vi "VibratomeGUI.vi"(8 "Error Out":errorcluster, 11 "Remote?":bool) -> ()   [LabVIEW 2014]
uses:
  Hardware/Table Stage/Controls/Translation Stage Cluster.ctl
  Controls/Translation Stage Types.ctl
  Controls/Translation Stage Quick Status.ctl
  Controls/Translation Stage Quick Controls.ctl
  Controls/QueueNames.ctl
  Controls/Queue Manager Actions.ctl
  Controls/MessagePacket.ctl
  <vilib>/Utility/miscctls.llb/LVPointTypeDef.ctl
  Hardware/Table Stage/Controls/Motion Translation Module Control.ctl
  Controls/Set Get Controls.ctl
  Controls/FGV Actions.ctl
panel:
  in  "Z STEP MOTION":enum16{"Fine", "Course", "Extra Course"}(ring)
  in  "Stop Button":bool
  in  "Slice":bool
  in  "Vibratome Controls":T1
  out "Message":string
  in  "Z Ctrl":T2
  out "Z Status":T3
  in  "Y Ctrl":T2
  out "Y Status":T3
  in  "X Ctrl":T2
  out "X Status":T3
  in  "XY STEP MOTION":enum16{"Fine", "Course", "Extra Course"}(ring)
  out "Cluster":cluster{"X":T4, "Y":T4, "Z":T4}
  in  "Exit":bool
  out "Processor Error Out":errorcluster
  out "GUI Error Out":errorcluster
  # "Vibratome Controls"
  # "Z Axis"
  # "Y Axis"
  # "X Axis"
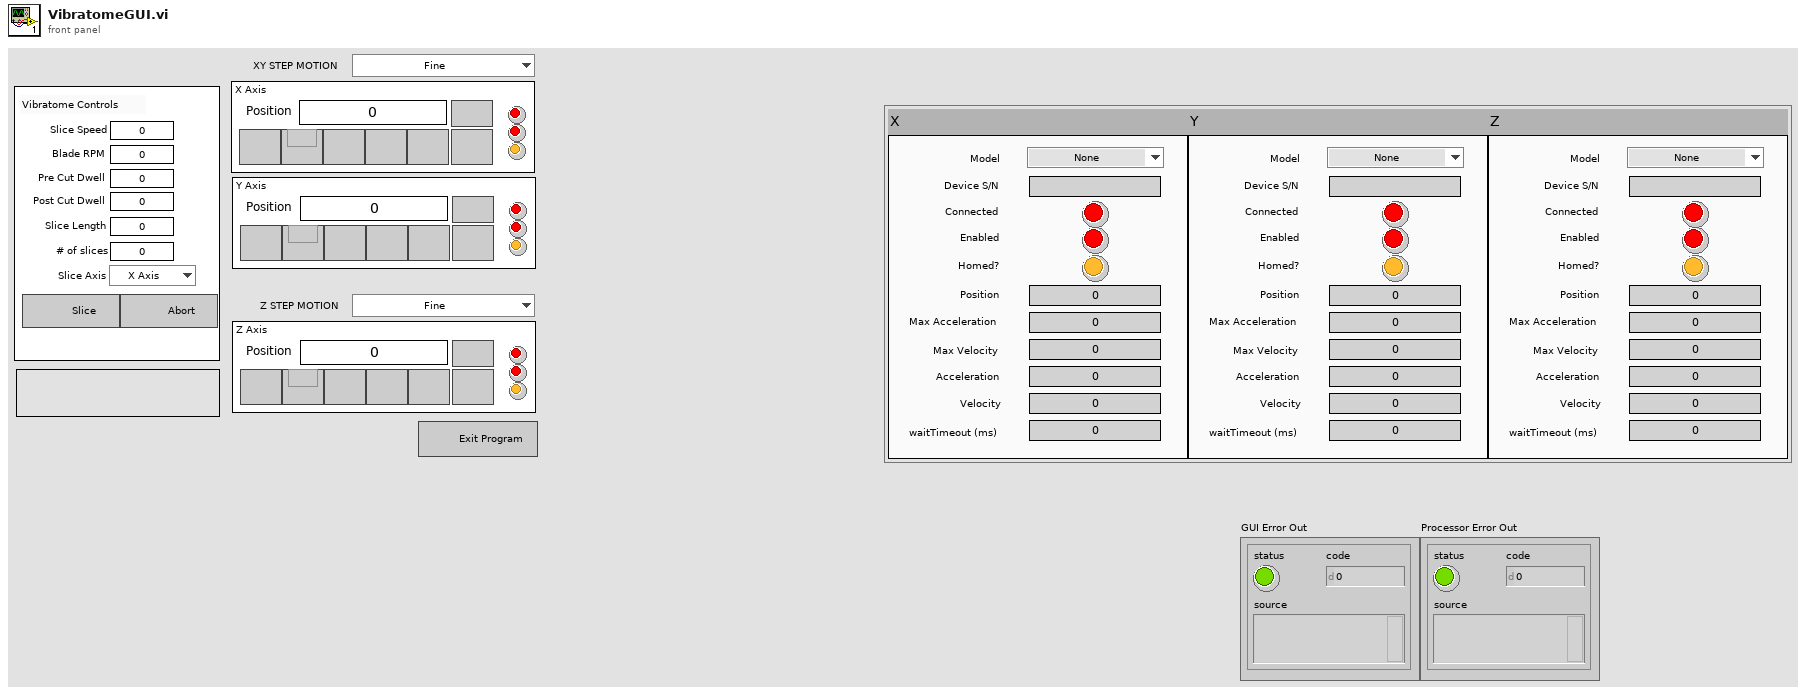
[diagram p1: front panel]
types:
  T1 = cluster{"Pre Cut Dwell":dbl, "Blade RPM":u16, "Slice Speed":dbl, "Post Cut Dwell":dbl, "Slice Length":dbl, "# of slices":dbl, "Slice Axis":enum16{"X Axis", "Y Axis", "Z Axis"}}
  T2 = typedef "Translation Stage Quick Controls.ctl" = cluster{"Position":dbl, "Next Button":bool, "Last Button":bool, "Previous Button":bool, "First Button":bool, "Home Button":bool, "Go":bool, "Settings Button":bool}
  T3 = typedef "Translation Stage Quick Status.ctl" = cluster{"Is.Enabled?":bool, "Is.Connected?":bool, "Is.Homed?":bool}
  T4 = typedef "Translation Stage Cluster.ctl" = cluster{"Position":dbl, "Is.Enabled?":bool, "Is.Connected?":bool, "Device SN":string, "AccelerationMaximum":dbl, "VelocityMaximum":dbl, "Acceleration":dbl, "Velocity":dbl, "waitTimeout (ms)":i32, "Model":T5, "Is.Homed?":bool}
  T5 = typedef "Translation Stage Types.ctl" = enum16{"None", "Thorlabs LTS", "Thorlabs MLJ"}
  T6 = typedef "MessagePacket.ctl" = cluster{"Message":string, "Parameter":variant}
  T7 = typedef "Queue Manager Actions.ctl" = enum16{"Init", "Enqueue", "Enqueue All", "Preview Queue", "Dequeue", "Get Status", "Flush Queue", "Flush All Queues", "Release All Queues", "Release Queue", "Enqueue at Opposite End"}
  T8 = typedef "QueueNames.ctl" = enum16{"Main GUI", "Main Scan Processor", "Main Display", "Main Table Stage GUI", "Main Table Stage Proc.", "Scan Engine", "Vibratome GUI", "Vibratome Processor", "Slice Engine"}
  T9 = enum16{"Set Configuration", "Get Configuration", "Enable Motor", "Disable Motor", "Get Status", "Open Session", "Close Session", "Set Limits", "Get Limits"}
  T10 = typedef "FGV Actions.ctl" = enum16{"Init", "Set", "Get", "Clear"}
  T11 = typedef "Set Get Controls.ctl" = enum16{"Set", "Get"}
  T12 = typedef "Motion Translation Module Control.ctl" = enum16{"Init", "Home", "Status", "Velocity/Accel", "Position", "Jog", "Stop", "Uninit", "Enable", "Disable"}
  T13 = cluster{"X Stage":T4, "Y Stage":T4, "Z Stage":T4}
  T14 = typedef "System Parameters.ctl" = cluster{"OCT":cluster{"Focal Length":dbl[unit]}, "Vibratome":cluster{"Z Bottom [mm]":dbl, "Pre Cut Dwell [s]":dbl, "Blade Frequency [RPM]":u16, "Slice Speed [mm/s]":dbl, "Post Cut Dwell [s]":dbl, "Ramp Time [s]":dbl, "Start X [mm]":dbl, "Start Y [mm]":dbl, "Slice Length [mm]":dbl, "Slice Axis":enum16{"X Axis", "Y Axis", "Z Axis"}, "Controller VISA Ref":refnum<visa-resource-name>}, "Table Stages":cluster{"X Stage":T4, "Y Stage":T4, "Z Stage":T4}}
  T15 = cluster{"Z Bottom [mm]":dbl, "Pre Cut Dwell [s]":dbl, "Blade Frequency [RPM]":u16, "Slice Speed [mm/s]":dbl, "Post Cut Dwell [s]":dbl, "Ramp Time [s]":dbl, "Start X [mm]":dbl, "Start Y [mm]":dbl, "Slice Length [mm]":dbl, "Slice Axis":enum16{"X Axis", "Y Axis", "Z Axis"}, "Controller VISA Ref":refnum<visa-resource-name>}
  T16 = enum32{"Invalid", "Default", "Floating", "Floating/Auto-Hide", "Modal"}
  T17 = enum32{"Invalid", "Standard", "Closed", "Hidden", "Minimized", "Maximized"}
  T18 = typedef "LVPointTypeDef.ctl" = cluster{"Horizontal":i16, "Vertical":i16}
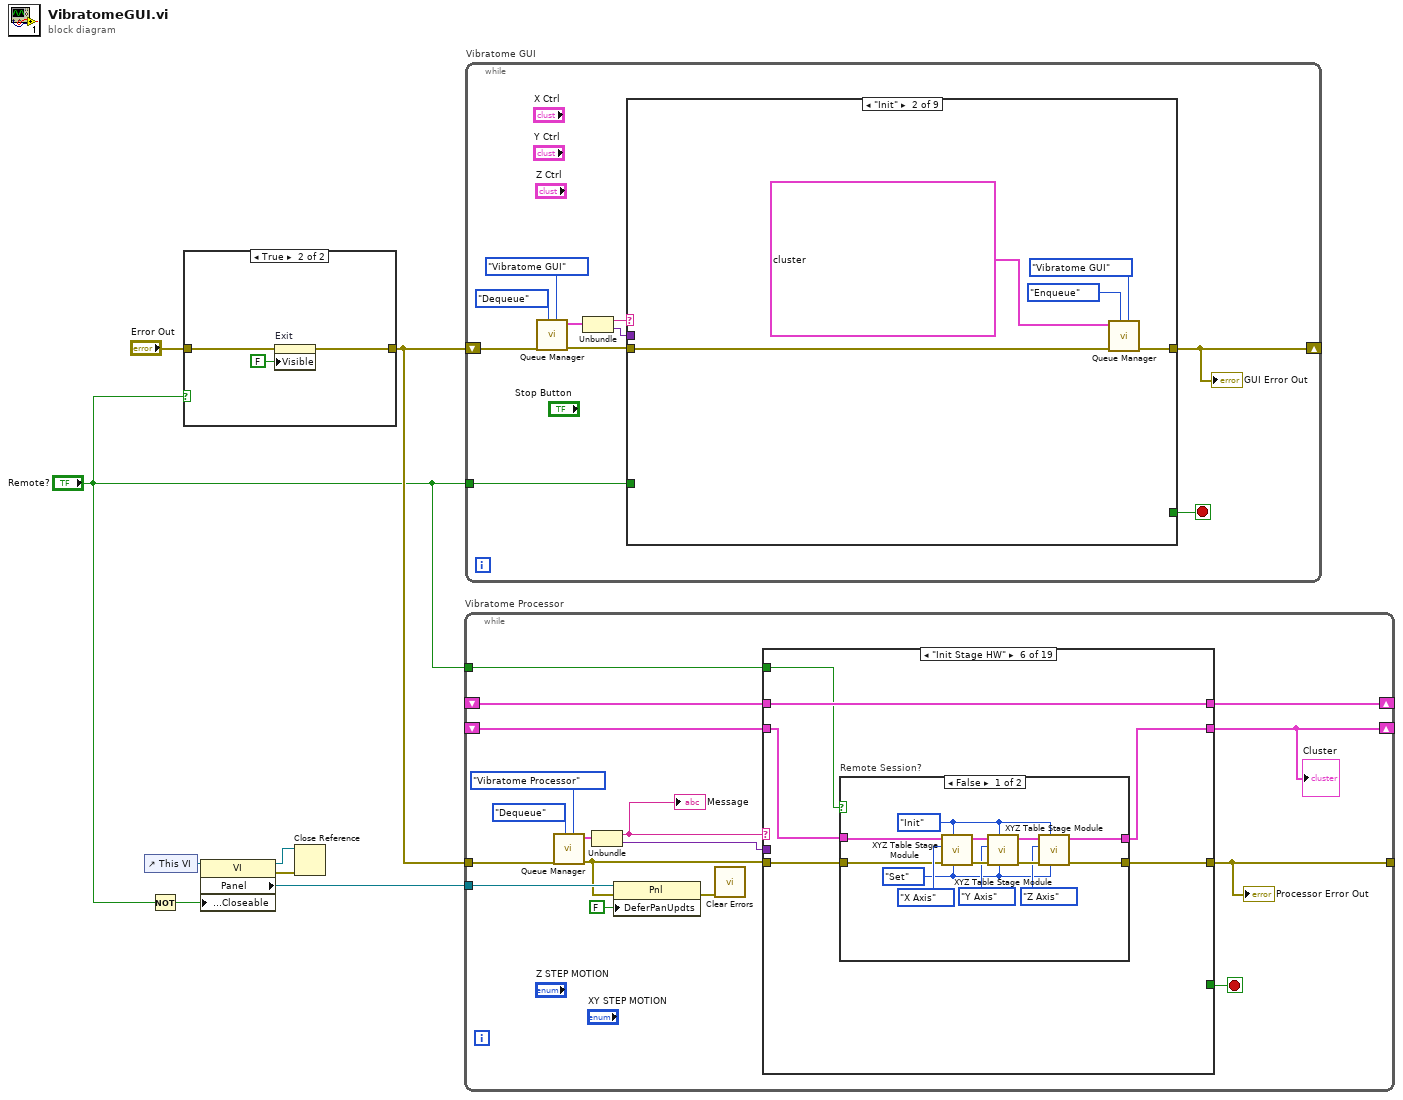
[diagram p0: block diagram]
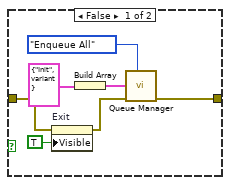
[diagram p2: hidden frame]
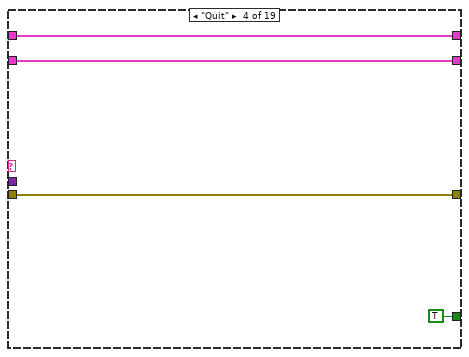
[diagram p6: hidden frame]
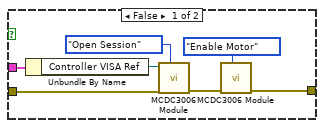
[diagram p10: hidden frame]
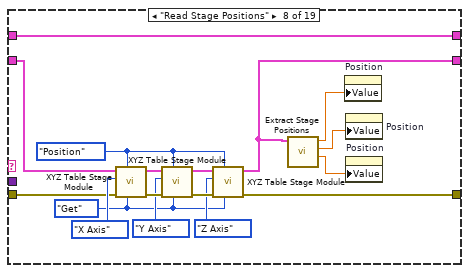
[diagram p11: hidden frame]
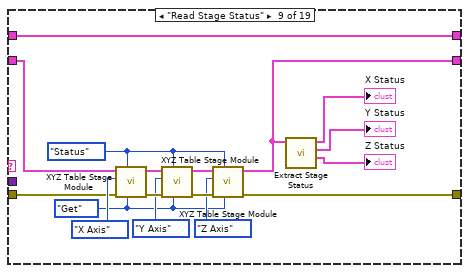
[diagram p12: hidden frame]
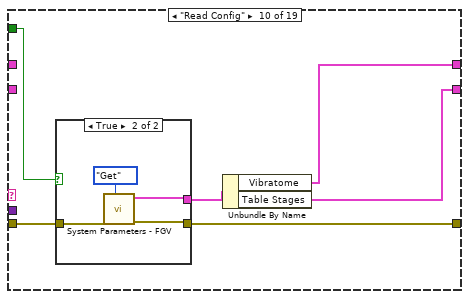
[diagram p13: hidden frame]
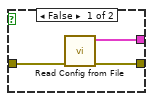
[diagram p14: hidden frame]
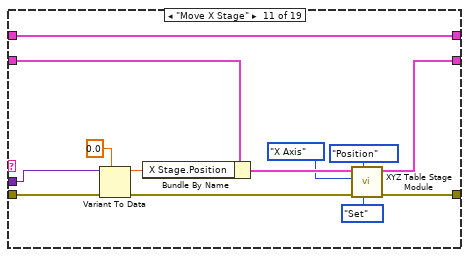
[diagram p15: hidden frame]
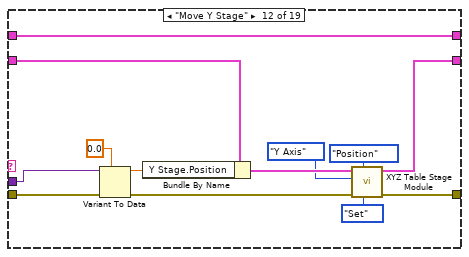
[diagram p16: hidden frame]
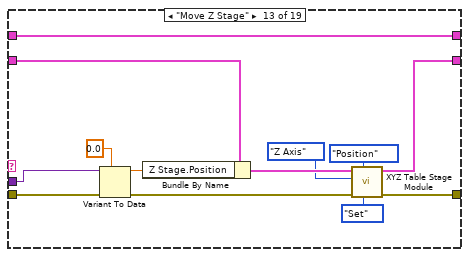
[diagram p17: hidden frame]
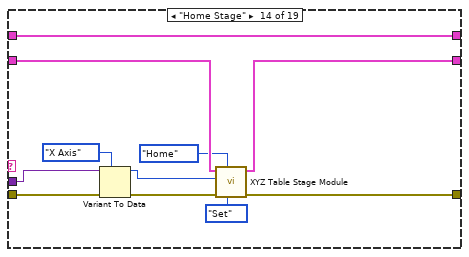
[diagram p18: hidden frame]
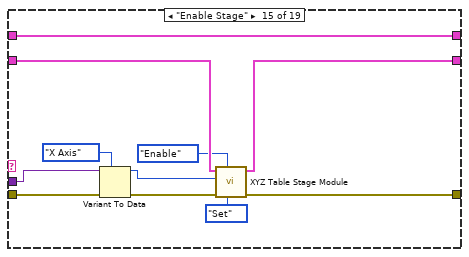
[diagram p19: hidden frame]
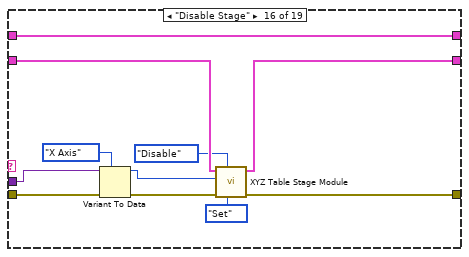
[diagram p20: hidden frame]
diagram:
  n1 = control-ref of="This VI"() -> (w7:refnum<vi>)
  n2 = Not(x="Remote?") -> (.not. x?=w1:bool)
  n3 = case shown="True" "Remote?" {
    tunnel: [w12 w17] -> w8
    tunnel: "Error Out" -> [w10 w18]
    frame False {
      n4 = property on="Exit" class="Bool"(error in=w10, "Visible"=TRUE) -> (error out=w9:errorcluster)  [unwired: 1 in, 1 out]
      n5 = Build Array(T6 {"Message"="Init", "Parameter"=variant} ("Message Packet [In]")) -> (w13:T6[])
      n6 = call "Queue Manager.vi"("Action"=Queue_Manager_Actions."Enqueue All", "Error In"=w9, "Message Packet Array"=w13) -> ("Error Out"=w12:errorcluster)  [unwired: 4 in, 4 out]
    }
    frame True {
      n7 = property on="Exit" class="Bool"(error in=w18, "Visible"=FALSE) -> (error out=w17:errorcluster)  [unwired: 1 in, 1 out]
    }
  }
  n8 = property class="VI"(reference=w7, "Front Panel.Closeable"=w1) -> (reference out=w5:refnum<vi>, error out=w6:errorcluster, "Panel"=w4:refnum<vi>)  [unwired: 1 in]
  n9 = Close Reference(reference=w5, error in (no error)=w6) -> ()  [unwired: 1 out]
  n10 = while "Vibratome Processor" {
    tunnel: w8 -> [w33]
    tunnel: [w35] -> _
    shift-right: [w24] -> _
    shift-left: _ -> [w27]
    shift-right: [w26] -> _
    shift-left: _ -> [w25]
    tunnel: w4 -> [w23]
    tunnel: "Remote?" -> [w19]
    stop <- w29 stop-if-true
    n11 = call "Queue Manager.vi"("Queue Name"=QueueNames."Vibratome Processor", "Action"=Queue_Manager_Actions."Dequeue", "Error In"=w33) -> ("Error Out"=w21:errorcluster, "Message Packet [Out]"=w32:T6)  [unwired: 4 in, 3 out]
    n12 = Unbundle(w32) -> ("Message"=w31:string, "Parameter"=w30:variant)
    "Message" <- w31
    n13 = property class="Pnl"(reference=w23, error in=w21, "DeferPanUpdts"=FALSE ("Defer Panel Updates")) -> (error out=w20:errorcluster)  [unwired: 1 out]
    n14 = call <vilib>:"Clear Errors.vi"("error in (no error)"=w20) -> ()  [unwired: 5 in, 2 out]
    n15 = case shown="\"Init Stage HW\"" w31 {
      tunnel: w21 -> [w38 w41 w42 w46 w49 w54 w74 w90 w107 w123 w143 w156 w169 w180 w191 w202 w207 w213 w233]
      tunnel: [w38 w41 w42 w46 w49 w55 w72 w98 w115 w121 w142 w155 w168 w179 w190 w201 w206 w212 w217] -> w35
      tunnel: w30 -> [_ _ _ _ _ _ _ _ _ _ w140 w153 w166 w177 w188 w199 _ _ _]
      tunnel: [_ _ _ TRUE _ _ _ _ _ _ _ _ _ _ _ _ _ _ _] -> w29
      tunnel: [w37 w40 w44 w48 _ w51 w75 w84 w105 w122 w139 w152 w165 w173 w184 w195 w204 w214 w226] -> w24
      tunnel: w27 -> [w37 w40 w44 w48 _ w53 w75 w89 w106 _ w135 w148 w161 w174 w185 w196 w204 w214 w229]
      tunnel: [w36 w39 w43 w47 _ w52 w73 w88 w101 w120 w131 w144 w157 w170 w181 w192 w208 w215 w220] -> w26
      tunnel: w25 -> [w36 w39 w43 w47 _ w52 w73 w88 w101 _ w131 w144 w157 w170 w181 w192 w208 w215 w220]
      tunnel: w19 -> [_ _ _ _ _ w50 w71 _ _ w118 _ _ _ _ _ _ _ _ _]
      frame "Unknown", Default {
      }
      frame "Finished Init" {
      }
      frame "Finished" {
      }
      frame "Quit" {
      }
      frame "Init" {
      }
      frame "Init Stage HW" {
        n16 = case "Remote Session?" shown="False" w50 {
          tunnel: [w66 w69] -> w55
          tunnel: w54 -> [w58 w69]
          tunnel: w53 -> [w57 w70]
          tunnel: [w56 w70] -> w51
          frame False {
            w59 = Set_Get_Controls."Set" ("Set/Get")
            w65 = Motion_Translation_Module_Control."Init" ("Action")
            n17 = call "XYZ Table Stage Module.vi"("Set/Get"=w59, "Action"=w65, "Error In"=w58, "Axis"=enum16{"X Axis", "Y Axis", "Z Axis"}."X Axis", "Table Stages"=w57) -> ("Error Out"=w68:errorcluster, "Table Stages Out"=w64:T13)  [unwired: 5 in]
            n18 = call "XYZ Table Stage Module.vi"("Set/Get"=w59, "Action"=w65, "Error In"=w68, "Axis"=enum16{"X Axis", "Y Axis", "Z Axis"}."Y Axis", "Table Stages"=w64) -> ("Error Out"=w67:errorcluster, "Table Stages Out"=w63:T13)  [unwired: 5 in]
            n19 = call "XYZ Table Stage Module.vi"("Set/Get"=w59, "Action"=w65, "Error In"=w67, "Axis"=enum16{"X Axis", "Y Axis", "Z Axis"}."Z Axis", "Table Stages"=w63) -> ("Error Out"=w66:errorcluster, "Table Stages Out"=w56:T13)  [unwired: 5 in]
          }
          frame True {
          }
        }
      }
      frame "Init Vibratome HW" {
        n20 = case "Remote Session?" shown="True" w71 {
          tunnel: w74 -> [w81 w83]
          tunnel: w73 -> [w79 _]
          tunnel: [w77 w83] -> w72
          frame False {
            n21 = Unbundle By Name(w79) -> ("Controller VISA Ref"=w78:refnum<visa-resource-name>)
            n22 = call "MCDC3006 Module.vi"("Actions"=T9."Open Session", "Error In"=w81, "VISA resource name"=w78) -> ("Error Out"=w80:errorcluster)  [unwired: 4 in, 4 out]
            n23 = call "MCDC3006 Module.vi"("Actions"=T9."Enable Motor", "Error In"=w80) -> ("Error Out"=w77:errorcluster)  [unwired: 5 in, 4 out]
          }
          frame True {
          }
        }
      }
      frame "Read Stage Positions" {
        w91 = Set_Get_Controls."Get" ("Set/Get")
        w97 = Motion_Translation_Module_Control."Position" ("Action")
        n24 = call "XYZ Table Stage Module.vi"("Set/Get"=w91, "Action"=w97, "Error In"=w90, "Axis"=enum16{"X Axis", "Y Axis", "Z Axis"}."X Axis", "Table Stages"=w89) -> ("Error Out"=w100:errorcluster, "Table Stages Out"=w96:T13)  [unwired: 5 in]
        n25 = call "XYZ Table Stage Module.vi"("Set/Get"=w91, "Action"=w97, "Error In"=w100, "Axis"=enum16{"X Axis", "Y Axis", "Z Axis"}."Y Axis", "Table Stages"=w96) -> ("Error Out"=w99:errorcluster, "Table Stages Out"=w95:T13)  [unwired: 5 in]
        n26 = call "XYZ Table Stage Module.vi"("Set/Get"=w91, "Action"=w97, "Error In"=w99, "Axis"=enum16{"X Axis", "Y Axis", "Z Axis"}."Z Axis", "Table Stages"=w95) -> ("Error Out"=w98:errorcluster, "Table Stages Out"=w84:T13)  [unwired: 5 in]
        n27 = call "Extract Stage Positions.vi"("Table Stages"=w84) -> ("Z Stage.Position"=w85:dbl, "Y Stage.Position"=w86:dbl, "X Stage.Position"=w87:dbl)  [unwired: 8 in]
        n28 = property on="Position" class="DigNum (strict)"("Value"=w87) -> ()  [unwired: 2 in, 2 out]
        n29 = property on="Position" class="DigNum (strict)"("Value"=w86) -> ()  [unwired: 2 in, 2 out]
        n30 = property on="Position" class="DigNum (strict)"("Value"=w85) -> ()  [unwired: 2 in, 2 out]
      }
      frame "Read Stage Status" {
        w108 = Set_Get_Controls."Get" ("Set/Get")
        w114 = Motion_Translation_Module_Control."Status" ("Action")
        n31 = call "XYZ Table Stage Module.vi"("Set/Get"=w108, "Action"=w114, "Error In"=w107, "Axis"=enum16{"X Axis", "Y Axis", "Z Axis"}."X Axis", "Table Stages"=w106) -> ("Error Out"=w117:errorcluster, "Table Stages Out"=w113:T13)  [unwired: 5 in]
        n32 = call "XYZ Table Stage Module.vi"("Set/Get"=w108, "Action"=w114, "Error In"=w117, "Axis"=enum16{"X Axis", "Y Axis", "Z Axis"}."Y Axis", "Table Stages"=w113) -> ("Error Out"=w116:errorcluster, "Table Stages Out"=w112:T13)  [unwired: 5 in]
        n33 = call "XYZ Table Stage Module.vi"("Set/Get"=w108, "Action"=w114, "Error In"=w116, "Axis"=enum16{"X Axis", "Y Axis", "Z Axis"}."Z Axis", "Table Stages"=w112) -> ("Error Out"=w115:errorcluster, "Table Stages Out"=w105:T13)  [unwired: 5 in]
        n34 = call "Extract Stage Status.vi"("Table Stages"=w105) -> ("Z Stage"=→"Z Status":T3, "Y Stage"=→"Y Status":T3, "X Stage"=→"X Status":T3)  [unwired: 8 in]
      }
      frame "Read Config" {
        n35 = case shown="True" w118 {
          tunnel: w123 -> [w126 w129]
          tunnel: [w125 w128] -> w121
          tunnel: [w124 w127] -> w119
          frame False {
            n36 = call "Read Config from File.vi"("error in (no error)"=w126) -> ("error out"=w125:errorcluster, "System Parameters"=w124:T14)  [unwired: 9 in]
          }
          frame True {
            n37 = call "System Parameters - FGV.vi"("Actions"=FGV_Actions."Get", "Error In"=w129) -> ("Error Out"=w128:errorcluster, "System Parameters"=w127:T14)  [unwired: 8 in]
          }
        }
        n38 = Unbundle By Name(w119) -> ("Vibratome"=w120:T15, "Table Stages"=w122:T13)
      }
      frame "Move X Stage" {
        n39 = Variant To Data(error in=w143, type=0.0 ("Value"), Variant=w140) -> (data=w134:dbl, error out=w141:errorcluster)
        n40 = Bundle By Name(cluster=w135, "X Stage.Position"=w134) -> (w133:T13)
        n41 = call "XYZ Table Stage Module.vi"("Set/Get"=Set_Get_Controls."Set", "Action"=Motion_Translation_Module_Control."Position", "Error In"=w141, "Axis"=enum16{"X Axis", "Y Axis", "Z Axis"}."X Axis", "Table Stages"=w133) -> ("Error Out"=w142:errorcluster, "Table Stages Out"=w139:T13)  [unwired: 5 in]
      }
      frame "Move Y Stage" {
        n42 = Variant To Data(error in=w156, type=0.0 ("Value"), Variant=w153) -> (data=w147:dbl, error out=w154:errorcluster)
        n43 = Bundle By Name(cluster=w148, "Y Stage.Position"=w147) -> (w146:T13)
        n44 = call "XYZ Table Stage Module.vi"("Set/Get"=Set_Get_Controls."Set", "Action"=Motion_Translation_Module_Control."Position", "Error In"=w154, "Axis"=enum16{"X Axis", "Y Axis", "Z Axis"}."Y Axis", "Table Stages"=w146) -> ("Error Out"=w155:errorcluster, "Table Stages Out"=w152:T13)  [unwired: 5 in]
      }
      frame "Move Z Stage" {
        n45 = Variant To Data(error in=w169, type=0.0 ("Value"), Variant=w166) -> (data=w160:dbl, error out=w167:errorcluster)
        n46 = Bundle By Name(cluster=w161, "Z Stage.Position"=w160) -> (w159:T13)
        n47 = call "XYZ Table Stage Module.vi"("Set/Get"=Set_Get_Controls."Set", "Action"=Motion_Translation_Module_Control."Position", "Error In"=w167, "Axis"=enum16{"X Axis", "Y Axis", "Z Axis"}."Z Axis", "Table Stages"=w159) -> ("Error Out"=w168:errorcluster, "Table Stages Out"=w165:T13)  [unwired: 5 in]
      }
      frame "Home Stage" {
        n48 = Variant To Data(error in=w180, type=enum16{"X Axis", "Y Axis", "Z Axis"}."X Axis" ("Axis"), Variant=w177) -> (data=w175:enum16{"X Axis", "Y Axis", "Z Axis"}, error out=w178:errorcluster)
        n49 = call "XYZ Table Stage Module.vi"("Set/Get"=Set_Get_Controls."Set", "Action"=Motion_Translation_Module_Control."Home", "Error In"=w178, "Axis"=w175, "Table Stages"=w174) -> ("Error Out"=w179:errorcluster, "Table Stages Out"=w173:T13)  [unwired: 5 in]
      }
      frame "Enable Stage" {
        n50 = Variant To Data(error in=w191, type=enum16{"X Axis", "Y Axis", "Z Axis"}."X Axis" ("Axis"), Variant=w188) -> (data=w186:enum16{"X Axis", "Y Axis", "Z Axis"}, error out=w189:errorcluster)
        n51 = call "XYZ Table Stage Module.vi"("Set/Get"=Set_Get_Controls."Set", "Action"=Motion_Translation_Module_Control."Enable", "Error In"=w189, "Axis"=w186, "Table Stages"=w185) -> ("Error Out"=w190:errorcluster, "Table Stages Out"=w184:T13)  [unwired: 5 in]
      }
      frame "Disable Stage" {
        n52 = Variant To Data(error in=w202, type=enum16{"X Axis", "Y Axis", "Z Axis"}."X Axis" ("Axis"), Variant=w199) -> (data=w197:enum16{"X Axis", "Y Axis", "Z Axis"}, error out=w200:errorcluster)
        n53 = call "XYZ Table Stage Module.vi"("Set/Get"=Set_Get_Controls."Set", "Action"=Motion_Translation_Module_Control."Disable", "Error In"=w200, "Axis"=w197, "Table Stages"=w196) -> ("Error Out"=w201:errorcluster, "Table Stages Out"=w195:T13)  [unwired: 5 in]
      }
      frame "Slice" {
        n54 = call "Extract Vibratome.vi"("Vibratome Controls"="Vibratome Controls", "Vibratome"=w208) -> ("Vibratome Out"=w205:T15)  [unwired: 9 in]
        n55 = call "Slice Module.vi"("Error In"=w207, "Table Stages"=w204, "Vibratome"=w205) -> ("Error Out"=w206:errorcluster)  [unwired: 6 in, 2 out]
      }
      frame "Exit" {
        n56 = call "Queue Manager.vi"("Queue Name"=QueueNames."Vibratome Processor", "Action"=Queue_Manager_Actions."Enqueue", "Error In"=w213, "Message Packet Array"=T6[] [{"Message"="Uninit", "Parameter"=variant}, {"Message"="Quit", "Parameter"=variant}]) -> ("Error Out"=w212:errorcluster)  [unwired: 3 in, 4 out]
      }
      frame "Uninit" {
        w221 = Set_Get_Controls."Set" ("Set/Get")
        w225 = Motion_Translation_Module_Control."Uninit" ("Action")
        n57 = call "XYZ Table Stage Module.vi"("Set/Get"=w221, "Action"=w225, "Error In"=w233, "Axis"=enum16{"X Axis", "Y Axis", "Z Axis"}."X Axis", "Table Stages"=w229) -> ("Error Out"=w231:errorcluster, "Table Stages Out"=w228:T13)  [unwired: 5 in]
        n58 = call "XYZ Table Stage Module.vi"("Set/Get"=w221, "Action"=w225, "Error In"=w231, "Axis"=enum16{"X Axis", "Y Axis", "Z Axis"}."Y Axis", "Table Stages"=w228) -> ("Error Out"=w232:errorcluster, "Table Stages Out"=w227:T13)  [unwired: 5 in]
        n59 = call "XYZ Table Stage Module.vi"("Set/Get"=w221, "Action"=w225, "Error In"=w232, "Axis"=enum16{"X Axis", "Y Axis", "Z Axis"}."Z Axis", "Table Stages"=w227) -> ("Error Out"=w230:errorcluster, "Table Stages Out"=w226:T13)  [unwired: 5 in]
        n60 = call "MCDC3006 Module.vi"("Actions"=T9."Disable Motor", "Error In"=w230) -> ("Error Out"=w219:errorcluster)  [unwired: 5 in, 4 out]
        n61 = call "MCDC3006 Module.vi"("Actions"=T9."Close Session", "Error In"=w219) -> ("Error Out"=w217:errorcluster)  [unwired: 5 in, 4 out]
      }
    }
    "Processor Error Out" <- w35
    "Cluster" <- w24
  }
  n62 = while "Vibratome GUI" {
    shift-right: [w243] -> _
    shift-left: w8 -> [w241]
    tunnel: "Remote?" -> [w234]
    stop <- w236 stop-if-true
    n63 = call "Queue Manager.vi"("Queue Name"=QueueNames."Vibratome GUI", "Action"=Queue_Manager_Actions."Dequeue", "Error In"=w241) -> ("Error Out"=w240:errorcluster, "Message Packet [Out]"=w239:T6)  [unwired: 4 in, 3 out]
    n64 = Unbundle(w239) -> ("Message"=w238:string, "Parameter"=w237:variant)
    n65 = case shown="\"Init\"" w238 {
      tunnel: w240 -> [w244 w245 w250 w251 w253 w257 w260 w333 w345]
      tunnel: [w244 w246 w250 w251 w252 w257 w259 w334 w345] -> w243
      tunnel: w237 -> [_ _ _ _ _ _ _ _ _]
      tunnel: [_ _ _ _ _ _ _ _ TRUE] -> w236
      tunnel: w234 -> [_ _ _ _ _ _ w258 w328 _]
      frame "Unknown", Default {
      }
      frame "Init" {
        n66 = call "Queue Manager.vi"("Queue Name"=QueueNames."Vibratome GUI", "Action"=Queue_Manager_Actions."Enqueue", "Error In"=w245, "Message Packet Array"=T6[] [{"Message"="Init Variables", "Parameter"=variant}, {"Message"="Set Front Panel", "Parameter"=variant}, {"Message"="Load User Settings", "Parameter"=variant}, {"Message"="Configure Hardware", "Parameter"=variant}, {"Message"="Wait for Complete", "Parameter"=variant}, {"Message"="Wait for User Input", "Parameter"=variant}]) -> ("Error Out"=w246:errorcluster)  [unwired: 3 in, 4 out]
      }
      frame "Init Variables" {
      }
      frame "Load User Settings" {
      }
      frame "Configure Hardware" {
        n67 = call "Queue Manager.vi"("Queue Name"=QueueNames."Vibratome Processor", "Action"=Queue_Manager_Actions."Enqueue", "Error In"=w253, "Message Packet Array"=T6[] [{"Message"="Read Config", "Parameter"=variant}, {"Message"="Init Stage HW", "Parameter"=variant}, {"Message"="Read Stage Status", "Parameter"=variant}, {"Message"="Read Stage Positions", "Parameter"=variant}, {"Message"="Init Vibratome HW", "Parameter"=variant}, {"Message"="Finished Init", "Parameter"=variant}]) -> ("Error Out"=w252:errorcluster)  [unwired: 3 in, 4 out]
      }
      frame "Wait for Complete" {
      }
      frame "Wait for User Input" {
        n68 = event shown="[1] Panel Close;  Application Instance Close;  \"Exit\": Value Change" {
          selector: _ -> [_ _ _ _ _ _]
          dyn-events: _ -> [_ _ _ _ _ _]
          timeout: _ -> [_ _ _ _ _ _]
          tunnel: w260 -> [w261 w264 w272 w294 w309 w324]
          tunnel: [w261 w263 w277 w281 w296 w311] -> w259
          tunnel: w258 -> [_ w262 _ _ _ _]
          event Timeout {
            n69 = event-data() -> ()  [unwired: 1 in, 3 out]
          }
          event Panel Close; Application Instance Close; "Exit": Value Change {
            n70 = event-data() -> ()  [unwired: 1 in, 3 out]
            n71 = case shown="True" w262 {
              tunnel: w264 -> [w268 w270]
              tunnel: [w267 w270] -> w263
              frame False {
                n72 = Build Array(T6 {"Message"="Exit", "Parameter"=variant} ("Message Packet [In]")) -> (w265:T6[])
                n73 = call "Queue Manager.vi"("Action"=Queue_Manager_Actions."Enqueue All", "Error In"=w268, "Message Packet Array"=w265) -> ("Error Out"=w267:errorcluster)  [unwired: 4 in, 4 out]
              }
              frame True {
              }
            }
          }
          event "Slice": Value Change {
            n74 = event-data() -> ()  [unwired: 1 in, 6 out]
            n75 = Build Array(T6 {"Message"="Wait for User Input", "Parameter"=variant} ("Message Packet [In]")) -> (w275:T6[])
            n76 = call "Queue Manager.vi"("Queue Name"=QueueNames."Vibratome GUI", "Action"=Queue_Manager_Actions."Enqueue", "Error In"=w272, "Message Packet Array"=w275) -> ("Error Out"=w277:errorcluster)  [unwired: 3 in, 4 out]
            n77 = call "Queue Manager.vi"("Queue Name"=QueueNames."Vibratome Processor", "Action"=Queue_Manager_Actions."Enqueue", "Error In"=w272, "Message Packet Array"=T6[] [{"Message"="Slice", "Parameter"=variant}, {"Message"="Finished", "Parameter"=variant}]) -> ()  [unwired: 3 in, 5 out]
          }
          event Value Change {
            n78 = event-data() -> ()  [unwired: 1 in, 1 out]
            n79 = property on="Position" class="DigNum (strict)"(error in=w294) -> (error out=w291:errorcluster, "Value"=w289:dbl)  [unwired: 1 in, 1 out]
            n80 = Bundle By Name(cluster=T6 {"Message"="Move X Stage", "Parameter"=variant} ("Message Packet [In]"), "Parameter"=w289) -> (w288:T6)
            n81 = Build Array(w288, T6 {"Message"="Finished", "Parameter"=variant} ("Message Packet [In]")) -> (w287:T6[])
            n82 = call "Queue Manager.vi"("Queue Name"=QueueNames."Vibratome Processor", "Action"=Queue_Manager_Actions."Enqueue", "Error In"=w291, "Message Packet Array"=w287) -> ("Error Out"=w282:errorcluster)  [unwired: 3 in, 4 out]
            n83 = Build Array(T6 {"Message"="Wait for User Input", "Parameter"=variant} ("Message Packet [In]")) -> (w283:T6[])
            n84 = call "Queue Manager.vi"("Queue Name"=QueueNames."Vibratome GUI", "Action"=Queue_Manager_Actions."Enqueue", "Error In"=w282, "Message Packet Array"=w283) -> ("Error Out"=w281:errorcluster)  [unwired: 3 in, 4 out]
          }
          event Value Change {
            n85 = event-data() -> ()  [unwired: 1 in, 1 out]
            n86 = property on="Position" class="DigNum (strict)"(error in=w309) -> (error out=w306:errorcluster, "Value"=w304:dbl)  [unwired: 1 in, 1 out]
            n87 = Bundle By Name(cluster=T6 {"Message"="Move Y Stage", "Parameter"=variant} ("Message Packet [In]"), "Parameter"=w304) -> (w303:T6)
            n88 = Build Array(w303, T6 {"Message"="Finished", "Parameter"=variant} ("Message Packet [In]")) -> (w302:T6[])
            n89 = call "Queue Manager.vi"("Queue Name"=QueueNames."Vibratome Processor", "Action"=Queue_Manager_Actions."Enqueue", "Error In"=w306, "Message Packet Array"=w302) -> ("Error Out"=w297:errorcluster)  [unwired: 3 in, 4 out]
            n90 = Build Array(T6 {"Message"="Wait for User Input", "Parameter"=variant} ("Message Packet [In]")) -> (w298:T6[])
            n91 = call "Queue Manager.vi"("Queue Name"=QueueNames."Vibratome GUI", "Action"=Queue_Manager_Actions."Enqueue", "Error In"=w297, "Message Packet Array"=w298) -> ("Error Out"=w296:errorcluster)  [unwired: 3 in, 4 out]
          }
          event Value Change {
            n92 = event-data() -> ()  [unwired: 1 in, 1 out]
            n93 = property on="Position" class="DigNum (strict)"(error in=w324) -> (error out=w321:errorcluster, "Value"=w319:dbl)  [unwired: 1 in, 1 out]
            n94 = Bundle By Name(cluster=T6 {"Message"="Move Z Stage", "Parameter"=variant} ("Message Packet [In]"), "Parameter"=w319) -> (w318:T6)
            n95 = Build Array(w318, T6 {"Message"="Finished", "Parameter"=variant} ("Message Packet [In]")) -> (w317:T6[])
            n96 = call "Queue Manager.vi"("Queue Name"=QueueNames."Vibratome Processor", "Action"=Queue_Manager_Actions."Enqueue", "Error In"=w321, "Message Packet Array"=w317) -> ("Error Out"=w312:errorcluster)  [unwired: 3 in, 4 out]
            n97 = Build Array(T6 {"Message"="Wait for User Input", "Parameter"=variant} ("Message Packet [In]")) -> (w313:T6[])
            n98 = call "Queue Manager.vi"("Queue Name"=QueueNames."Vibratome GUI", "Action"=Queue_Manager_Actions."Enqueue", "Error In"=w312, "Message Packet Array"=w313) -> ("Error Out"=w311:errorcluster)  [unwired: 3 in, 4 out]
          }
        }
      }
      frame "Set Front Panel" {
        n99 = Select(t=T17."Hidden" ("Front Panel Window:State"), s=w328, f=T17."Standard" ("Front Panel Window:State")) -> (s? t:f=w329:T17)
        n100 = control-ref of="This VI"() -> (w332:refnum<vi>)
        n101 = Select(t=T16."Default" ("Front Panel Window:Behavior"), s=w328, f=T16."Modal") -> (s? t:f=w325:T16)
        n102 = property class="VI"(reference=w332, error in=w333, "FP.State"=w329, "FP.Behavior"=w325) -> (error out=w336:errorcluster, "Panel"=w339:refnum<vi>)  [unwired: 1 out]
        n103 = property class="Pnl"(reference=w339, error in=w336) -> (error out=w337:errorcluster, "Panes[]"=w338:refnum<vi>[])  [unwired: 1 out]
        n104 = for {
          tunnel: w338 -> [w343] mode=indexing
          tunnel: w337 -> [w341]
          tunnel: [w340] -> w335 mode=indexing
          n105 = property class="Pane"(reference=w343, error in=w341, "Origin"=T18 {"Horizontal"=0, "Vertical"=0}) -> (error out=w340:errorcluster)  [unwired: 1 out]
        }
        n106 = Merge Errors(w335) -> (w334:errorcluster)
      }
      frame "Exit" {
      }
    }
    "GUI Error Out" <- w243
  }
